vi "Status pH.vi"(8 "error in (no error)":errorcluster, 11 "VISA Resource in":refnum<visa-resource-name>) -> (0 "error out":errorcluster, 2 "pH":dbl, 3 "VISA Resource out":refnum<visa-resource-name>)   [LabVIEW 2020, in "plugin_flodx_ph_probe.lvlib" / "mock_driver.lvlib"]
doc: "Emulates reading pH from the probe, but always returns 9.560."
uses:
  mock_driver.lvlib
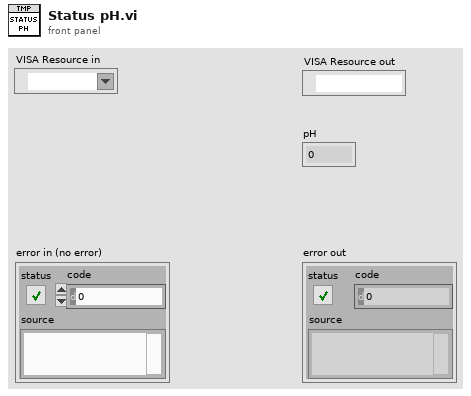
[diagram p1: front panel]
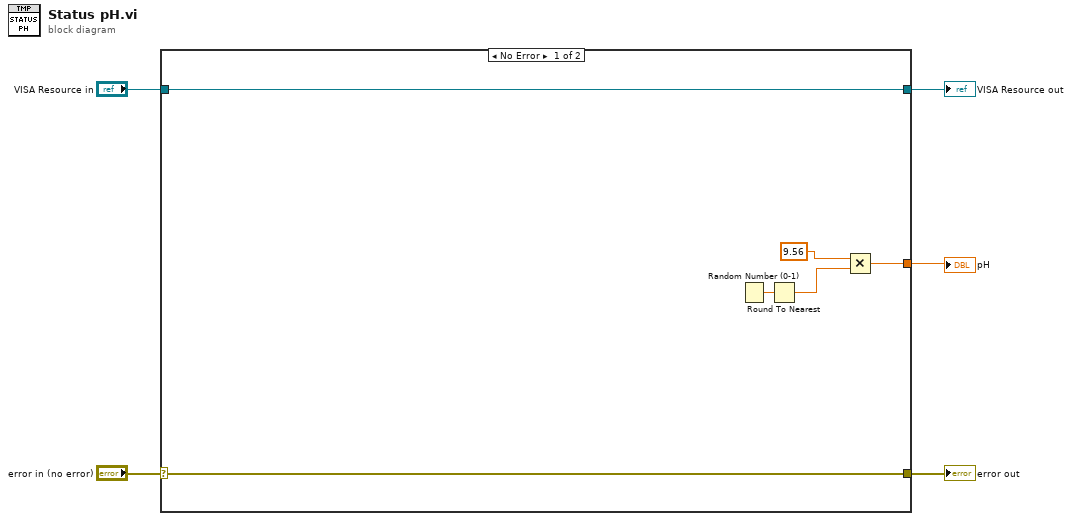
[diagram p0: block diagram]
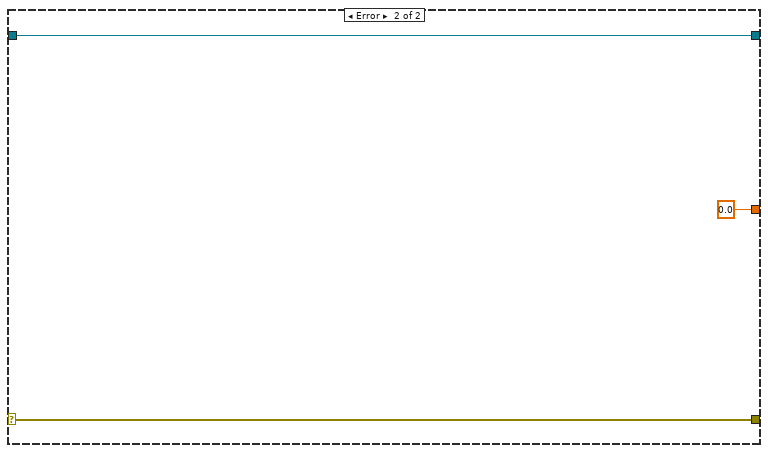
[diagram p2: hidden frame]
diagram:
  n1 = case shown="No Error" "error in (no error)" {
    selector: "error in (no error)" -> [w10 w13]
    tunnel: "VISA Resource in" -> [w11 w14]
    tunnel: [w11 w14] -> w4
    tunnel: [w10 w13] -> w2
    tunnel: [w8 0.0 ("pH")] -> w1
    frame No Error {
      n2 = Random Number (0-1)() -> (number: 0 to 1=w7:dbl)
      n3 = Round To Nearest(number=w7) -> (nearest integer value=w6:dbl)
      n4 = Multiply(x=9.56 ("pH"), y=w6) -> (x*y=w8:dbl)
    }
    frame Error {
    }
  }
  "VISA Resource out" <- w4
  "error out" <- w2
  "pH" <- w1
